vi "ADC_Tester.vi"() -> (5 "Plug in titles":string[](array[string]), 7 "Plug in values":string[](array[string]))   [LabVIEW 2010]
uses:
  Globals/Meas_global.vi
  Globals/Plug_in_data_global.vi
panel:
  in  "Index":i32
  out "Waveform Graph":dbl[](graph)
  out "% Change Factor":dbl[](array[numeric]) format="%.2f"
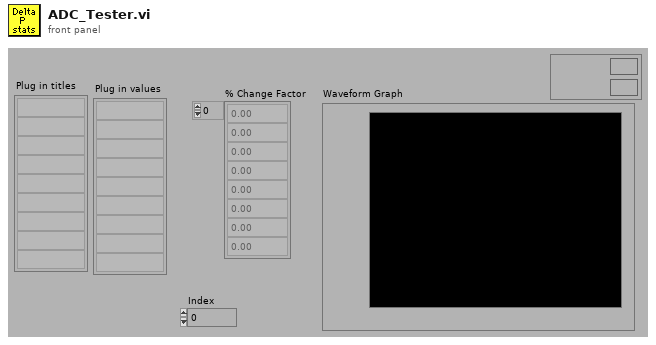
[diagram p1: front panel]
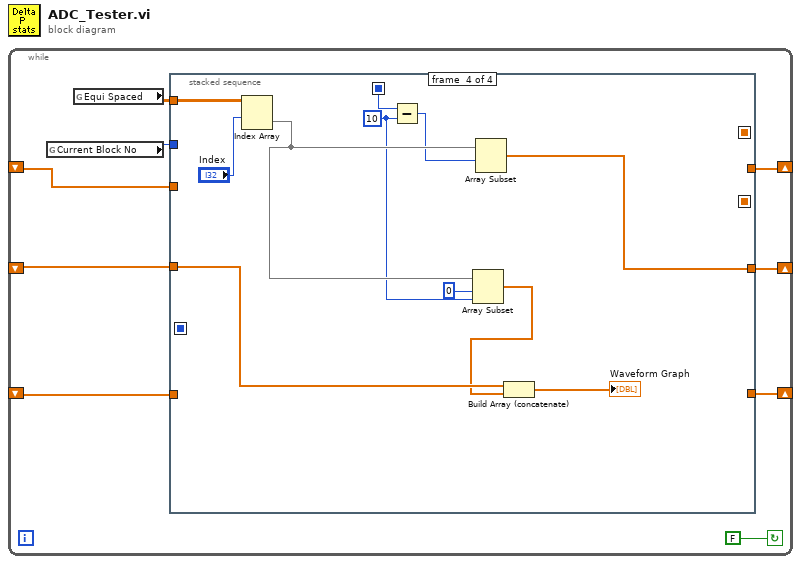
[diagram p0: block diagram]
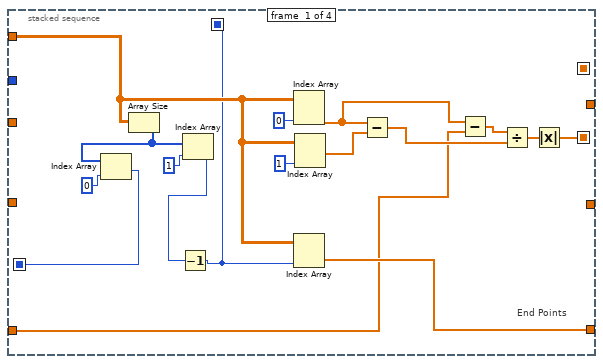
[diagram p2: hidden frame]
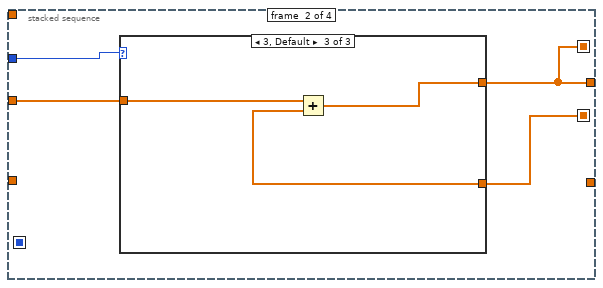
[diagram p3: hidden frame]
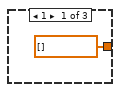
[diagram p4: hidden frame]
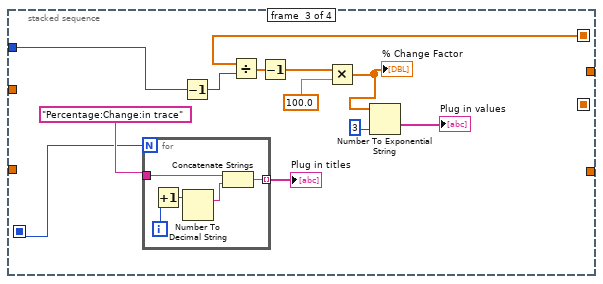
[diagram p6: hidden frame]
diagram:
  n1 = while {
    shift-left: _ -> [w2]
    shift-right: [w3] -> _
    shift-left: _ -> [w6]
    shift-right: [w5] -> _
    shift-left: _ -> [w4]
    shift-right: [w7] -> _
    stop <- FALSE continue-if-true
    n2 = global read "Meas_global.vi" "Current Block No"() -> (w8:i32)
    n3 = global read "Plug_in_data_global.vi" "Equi Spaced"() -> (w9:dbl[][])
    n4 = stacked-sequence {
      seq-local: [w16 _ _ _] -> [_ w27 _ _]
      seq-local: [_ w28 _ _] -> [_ _ w43 _]
      seq-local: [w13 _ _ _] -> [_ _ w40 _]
      seq-local: [w10 _ _ _] -> [_ _ _ w63]
      tunnel: w9 -> [w21 _ _ w59]
      tunnel: w8 -> [_ w30 w42 _]
      tunnel: [w12 _ _ _] -> w7
      tunnel: w6 -> [_ w29 _ _]
      tunnel: [_ w28 _ _] -> w5
      tunnel: w4 -> [w11 _ _ _]
      tunnel: [_ _ _ w62] -> w3
      tunnel: w2 -> [_ _ _ w61]
      frame #0 {
        # "End Points"
        n5 = Array Size(array=w21) -> (size(s)=w14:i32[])
        n6 = Index Array(array=w14, index=0 ("Index")) -> (element=w13:i32)
        n7 = Index Array(array=w14, index=1 ("Index")) -> (element=w23:i32)
        n8 = Decrement(x=w23) -> (x-1=w10:i32)
        n9 = Index Array(array=w21, index (col)=0 ("Index")) -> (element=w20:dbl[])  [unwired: 1 in]
        n10 = Index Array(array=w21, index (col)=w10) -> (element=w12:dbl[])  [unwired: 1 in]
        n11 = Index Array(array=w21, index (col)=1 ("Index")) -> (element=w22:dbl[])  [unwired: 1 in]
        n12 = Subtract(x=w20, y=w22) -> (x-y=w18:dbl[])
        n13 = Subtract(x=w20, y=w11) -> (x-y=w19:dbl[])
        n14 = Divide(x=w19, y=w18) -> (x/y=w17:dbl[])
        n15 = Absolute Value(x=w17) -> (abs(x)=w16:dbl[])
      }
      frame #1 {
        n16 = case shown="3, Default" w30 {
          tunnel: w29 -> [_ _ w35]
          tunnel: w27 -> [_ w32 w34]
          tunnel: [dbl[] [] w32 w33] -> w28
          frame 1 {
          }
          frame 2 {
          }
          frame 3, Default {
            n17 = Add(x=w35, y=w34) -> (x+y=w33:dbl[])
          }
        }
      }
      frame #2 {
        n18 = for {
          N: w40 -> [_]
          tunnel: "Percentage:Change:in trace" -> [w51]
          tunnel: [w48] -> w44 mode=indexing
          i -> [w52]
          n19 = Increment(x=w52) -> (x+1=w49:i32)
          n20 = Number To Decimal String(number=w49) -> (decimal integer string=w50:string)  [unwired: 1 in]
          n21 = Concatenate Strings(w51, w50) -> (w48:string)
        }
        "Plug in titles" <- w44
        n22 = Decrement(x=w42) -> (x-1=w41:i32)
        n23 = Divide(x=w43, y=w41) -> (x/y=w39:dbl[])
        n24 = Decrement(x=w39) -> (x-1=w36:dbl[])
        n25 = Multiply(x=w36, y=100.0) -> (x*y=w37:dbl[])
        "% Change Factor" <- w37
        n26 = Number To Exponential String(number=w37, precision (6)=3) -> (E-format string=→"Plug in values":string[])  [unwired: 2 in]
      }
      frame #3 {
        w55 = 10 ("y")
        n27 = Index Array(array=w59, index (row)="Index") -> (element=w58:dbl[])  [unwired: 1 in]
        n28 = Subtract(x=w63, y=w55) -> (x-y=w57:i32)
        n29 = Array Subset(array=w58, index=0 ("Array Index"), length=w55) -> (w54:dbl[])
        n30 = Array Subset(array=w58, index=w57) -> (w62:dbl[])  [unwired: 1 in]
        n31 = Build Array (concatenate)(w61, w54) -> (→"Waveform Graph":dbl[])
      }
    }
  }
